vi "Build Filename.vi"(9 "Test type":string, 10 "time stamp":timestamp, 11 "File config":T1) -> (3 "appended path":path)   [LabVIEW 2019]
panel:
  # "Build filename"
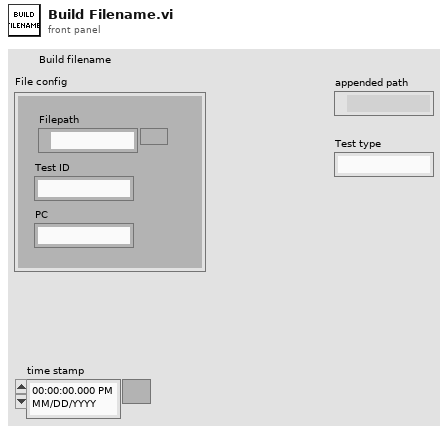
[diagram p1: front panel]
types:
  T1 = cluster{"Filepath":path, "Test ID":string, "PC":string}
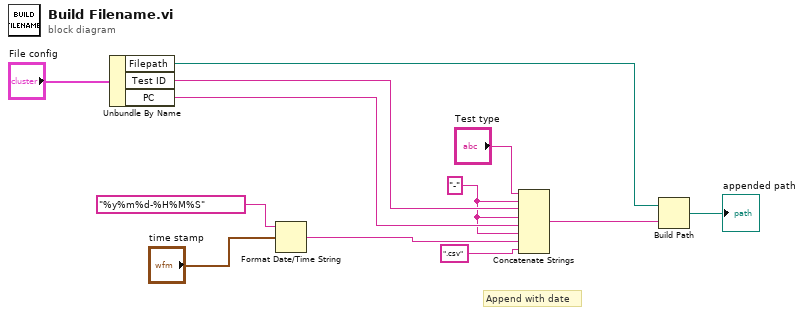
[diagram p0: block diagram]
diagram:
  w2 = "-" ("string")
  # "Append with date"
  n1 = Unbundle By Name("File config") -> ("Filepath"=w7:path, "Test ID"=w6:string, "PC"=w5:string)
  n2 = Format Date/Time String(time format string (%c)="%y%m%d-%H%M%S", seconds (now)="time stamp") -> (date/time string=w3:string)  [unwired: 1 in]
  n3 = Concatenate Strings("Test type", w2, w6, w2, w5, w2, w3, ".csv" ("Type")) -> (w12:string)
  n4 = Build Path(base path=w7, name or relative path=w12) -> (appended path=→"appended path":path)
